vi "Get Buffer Sizes.vi"(8 "error in (no error)":errorcluster, 11 "Buffers in":refnum<class "Buffers.lvclass">) -> (0 "error out":errorcluster, 1 "string buffer size":u64 format="%d bytes", 2 "engine buffer size":u64 format="%d bytes", 3 "Buffers out":refnum<class "Buffers.lvclass">)   [LabVIEW 2017, in "DSF Core.lvlib" / "Buffers.lvclass"]
uses:
  Buffers.lvclass
  Buffer/Buffer.lvclass
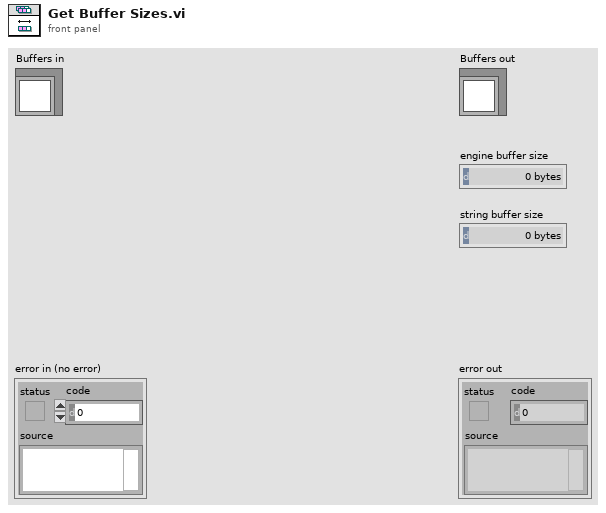
[diagram p1: front panel]
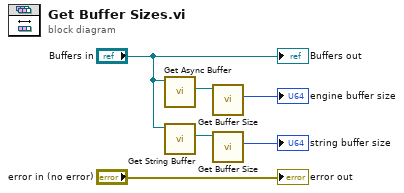
[diagram p0: block diagram]
diagram:
  n1 = call "Get Async Buffer.vi"("Buffers in"="Buffers in") -> ("Async Buffer"=w3:refnum<class "Buffer.lvclass">)  [unwired: 9 in, 1 out]
  n2 = call "Get String Buffer.vi"("Buffers in"="Buffers in") -> ("String Buffer"=w4:refnum<class "Buffer.lvclass">)  [unwired: 9 in, 1 out]
  n3 = call "Get Buffer Size.vi"("Buffer in"=w3) -> ("buffer size"=→"engine buffer size":u64)  [unwired: 9 in, 1 out]
  n4 = call "Get Buffer Size.vi"("Buffer in"=w4) -> ("buffer size"=→"string buffer size":u64)  [unwired: 9 in, 1 out]
  "error out" <- "error in (no error)"
  "Buffers out" <- "Buffers in"
